vi "Teleop.vi"(10 "Match Info":T1={"Autonomous Elapsed Seconds"=0.0, "TeleOp Elapsed Seconds"=0.0, "Disabled Elapsed Seconds"=0.0, "Visited Autonomous"=FALSE, "Visited TeleOp"=FALSE, "Visited Disabled"=FALSE, "Autonomous Settings"={"Autonomous Style"=enum."Independent", "VI Refnum"=refnum}}, 11 "Call Context":T2) -> ()   [LabVIEW 2020]
doc: "This VI is called for each TeleOp packet received from the DS where the robot is not disabled. It is often used to read from the joysticks and update I/O or to update setpoints for timed control loops. It should complete and return within 20 milliseconds or it may miss DS packets."
uses:
  <vilib>/Rock Robotics/WPI/DriverStation/WPI_DriverStationDerivedRobotMode.ctl
  <vilib>/Rock Robotics/WPI/DriverStation/WPI_DriverStationMatch Info.ctl
  <vilib>/Rock Robotics/WPI/Joystick/XBox Buttons Indexer.ctl
  <vilib>/Rock Robotics/WPI/Joystick/XBox Axes Indexer.ctl
  <vilib>/Rock Robotics/WPI/Relay/WPI_RelayValue.ctl
  <vilib>/Rock Robotics/Network Tables/NT Read Boolean.vi
  <vilib>/Rock Robotics/Network Tables/NT Read Number.vi
  Auxilary/AuxGlobals.vi
  Climb/ClimbGlobals.vi
  <vilib>/Rock Robotics/Network Tables/NT Write String.vi
  Human/HumanGlobal.vi
  DriveSystem/DriveGlobals.vi
  <vilib>/Rock Robotics/Network Tables/NT Write Number.vi
  <vilib>/Rock Robotics/Network Tables/NT Write Boolean.vi
  Vision/VisionGlobals.vi
  <vilib>/Rock Robotics/WPI/Joystick/WPI_JoystickArcadeMapping.vi
  <vilib>/Rock Robotics/WPI/ThirdParty/JAS_Junk/TrajLib/Trajectory_Library.lvlib
panel:
  out "Sample Slider 0":dbl(slide) scale=0.0..5.0
  out "Sample Boolean 1":bool
  out "Sample Boolean 0":bool
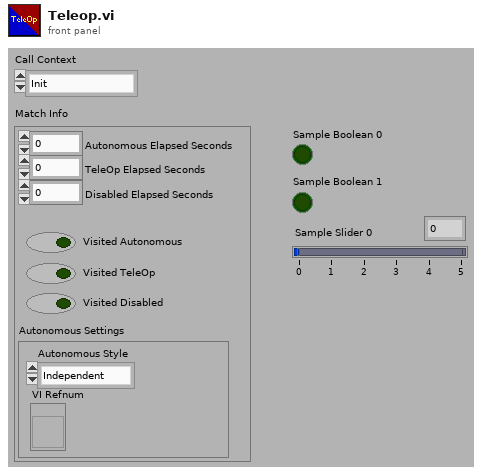
[diagram p1: front panel]
types:
  T1 = typedef "WPI_DriverStationMatch Info.ctl" = cluster{"Autonomous Elapsed Seconds":dbl, "TeleOp Elapsed Seconds":dbl, "Disabled Elapsed Seconds":dbl, "Visited Autonomous":bool, "Visited TeleOp":bool, "Visited Disabled":bool, "Autonomous Settings":cluster{"Autonomous Style":enum16{"Iterative", "Independent"}, "VI Refnum":refnum<vi>}}
  T2 = typedef "WPI_DriverStationDerivedRobotMode.ctl" = enum16{"Init", "Execute", "Stop"}
  T3 = typedef "XBox Buttons Indexer.ctl" = enum16{"A", "B", "X", "Y", "Left Bumper", "Right Bumper", "Back", "Start", "Left Joystick", "Right Joystick"}
  T4 = typedef "XBox Axes Indexer.ctl" = enum16{"Left X", "Left Y", "Left Trigger", "Right Trigger", "Right X", "Right Y"}
  T5 = typedef "WPI_RelayValue.ctl" = enum16{"Off", "On", "Forward", "Reverse"}
  T6 = typedef "WPI_RelayDevRef.ctl" = cluster{"DevStatus":errorcluster, "Relay Channel":T7, "Relay Direction":T8}
  T7 = typedef "FPGA_DIORelayChannel.ctl" = enum8{"Relay 0", "Relay 1", "Relay 2", "Relay 3", "Invalid"}
  T8 = typedef "WPI_RelayDirection.ctl" = enum16{"Both directions", "Forward only", "Reverse only"}
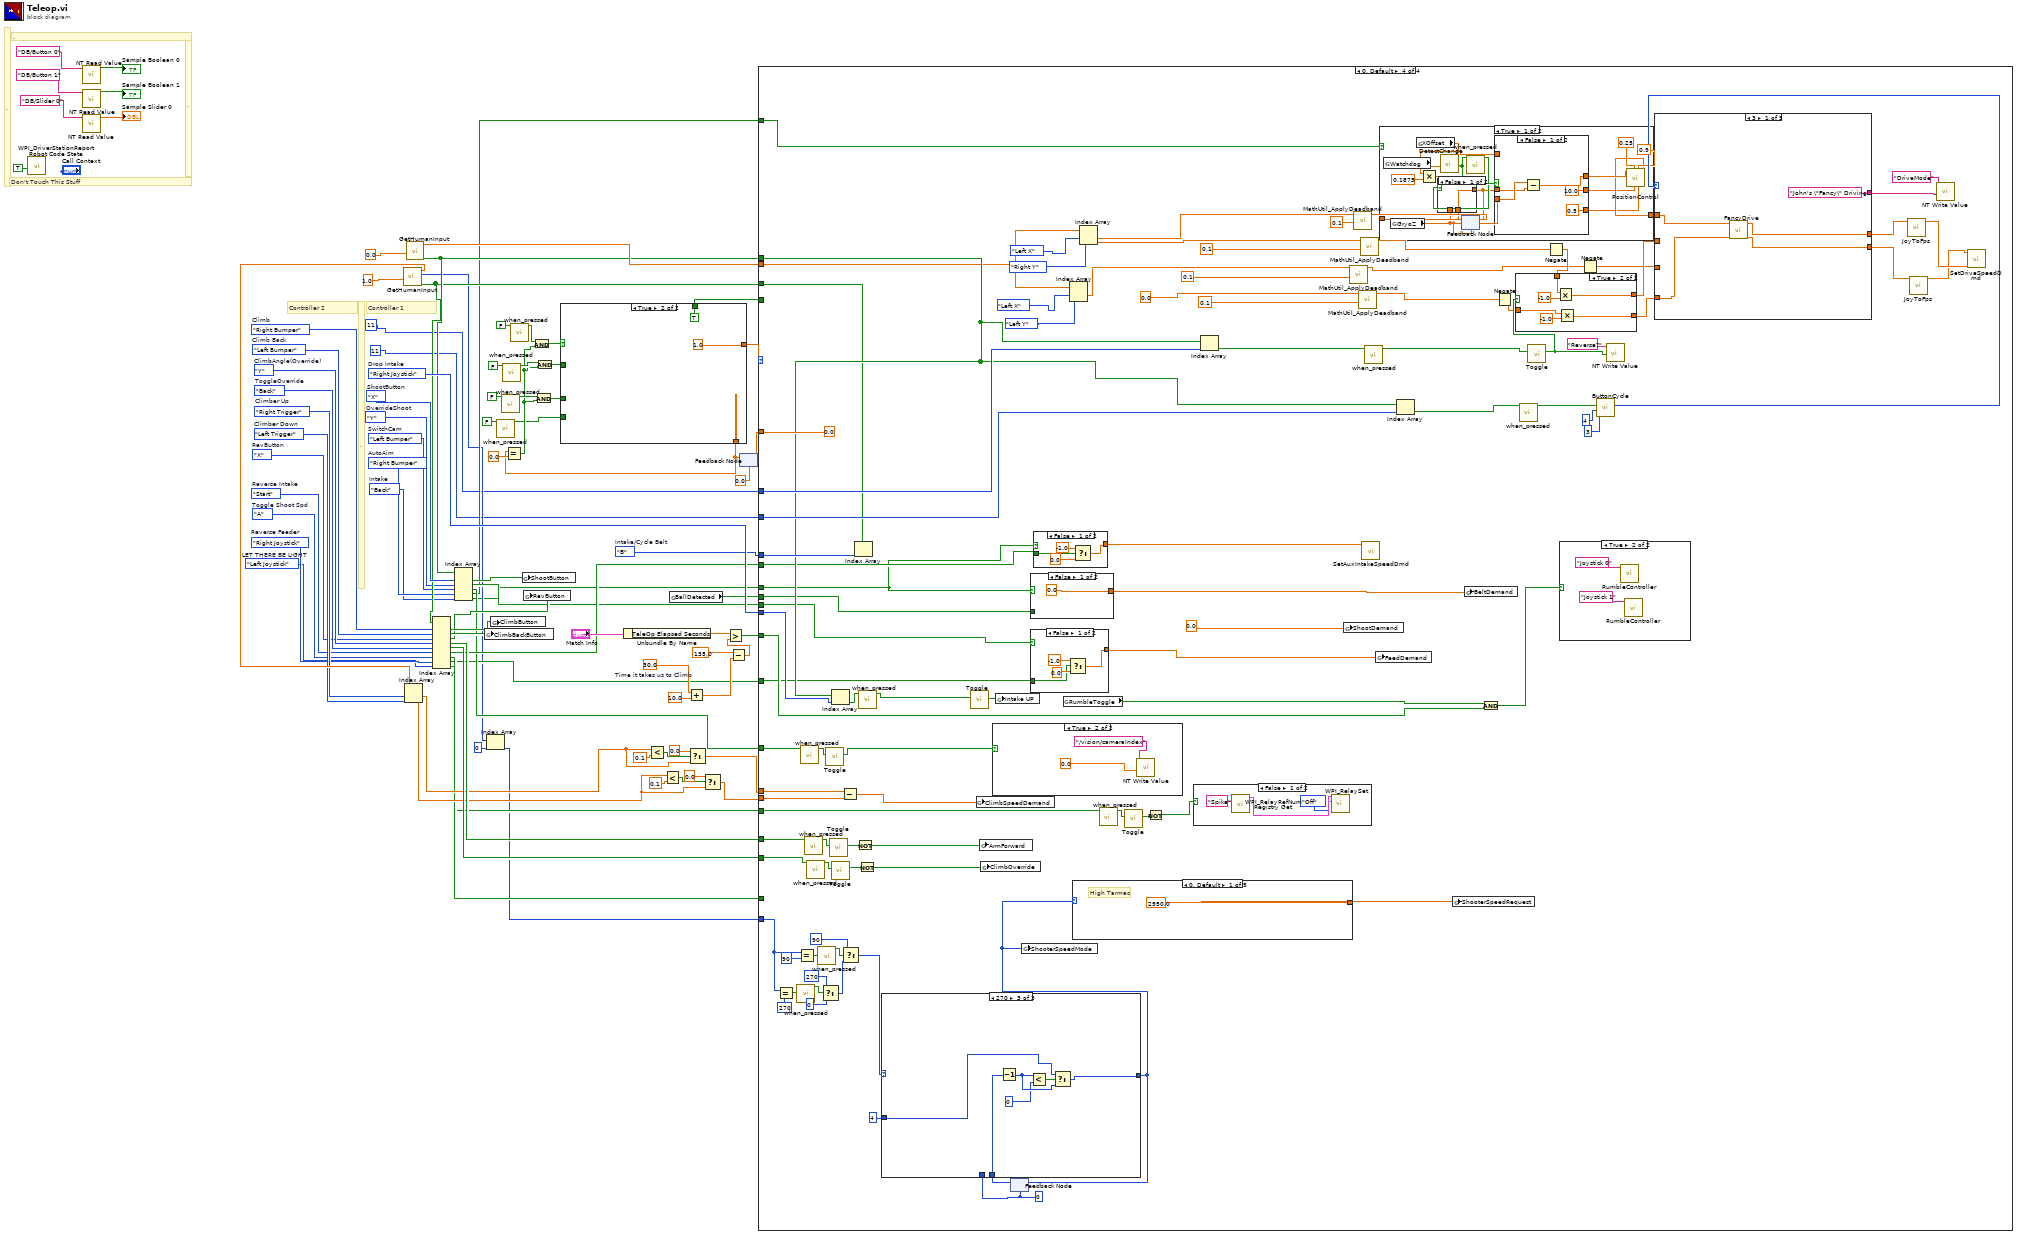
[diagram p0: block diagram]
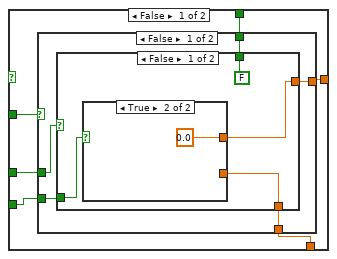
[diagram p2: hidden frame]
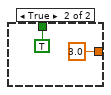
[diagram p4: hidden frame]
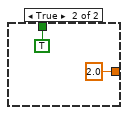
[diagram p5: hidden frame]
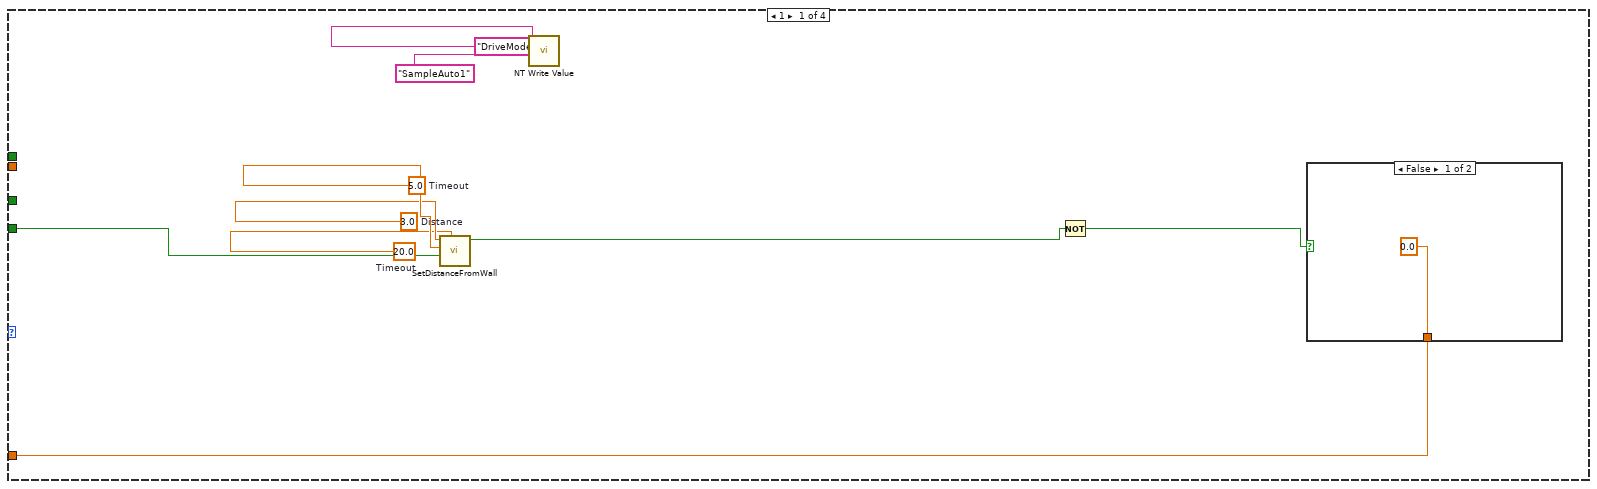
[diagram p6: hidden frame]
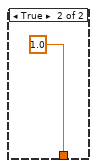
[diagram p7: hidden frame]
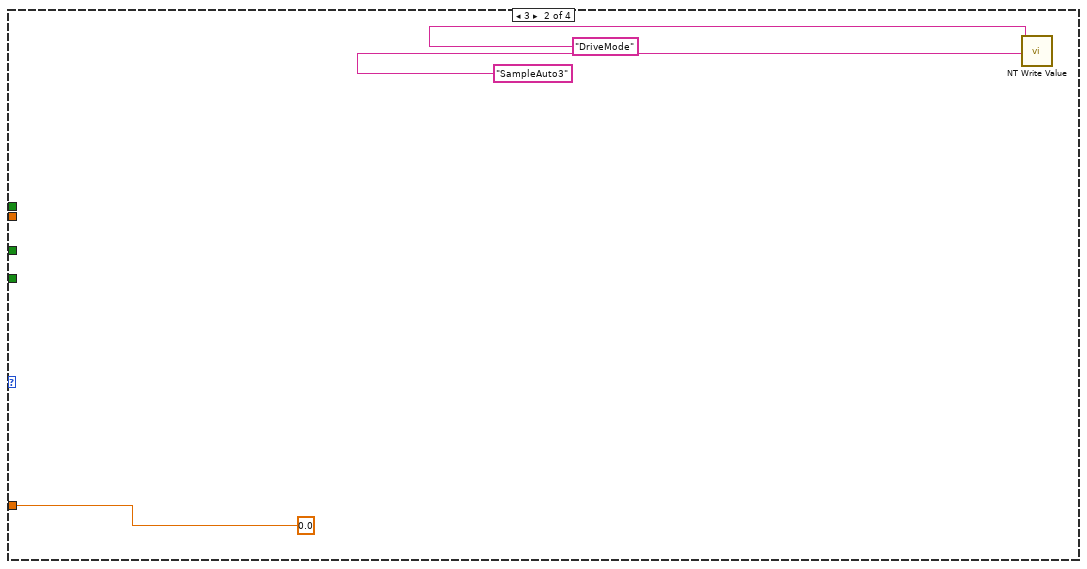
[diagram p8: hidden frame]
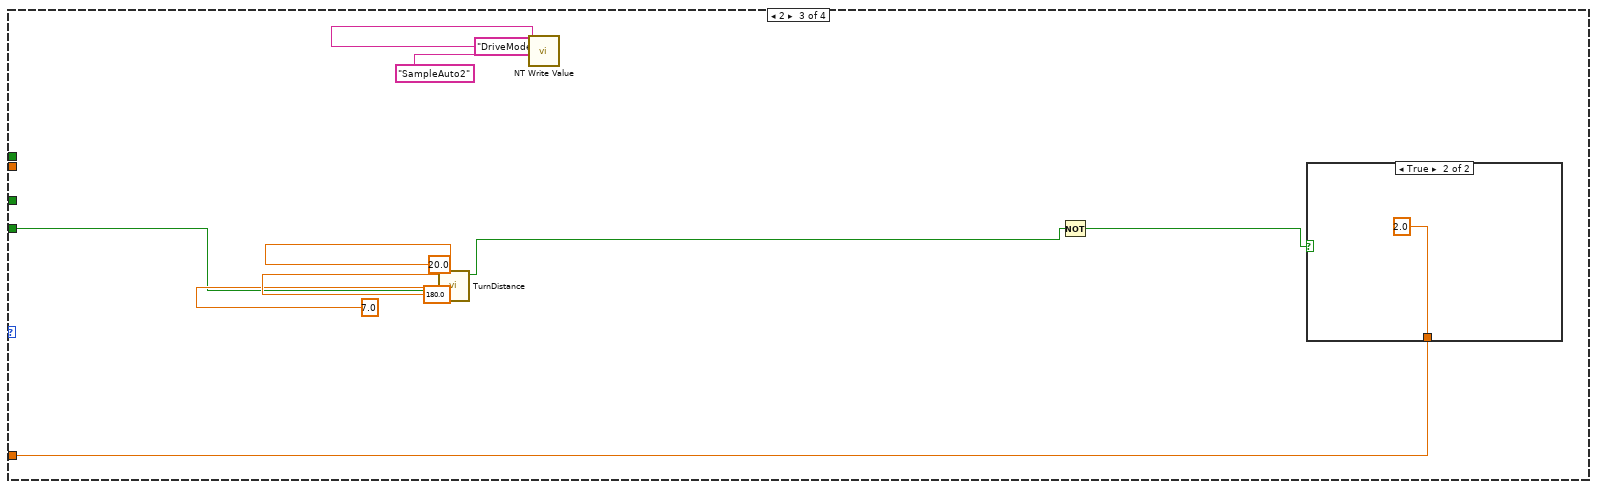
[diagram p9: hidden frame]
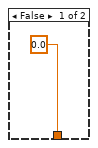
[diagram p10: hidden frame]
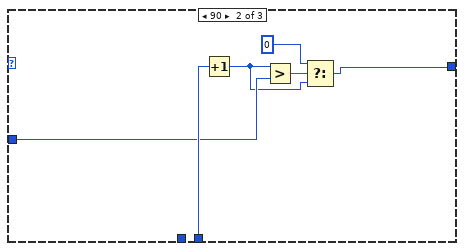
[diagram p12: hidden frame]
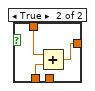
[diagram p13: hidden frame]
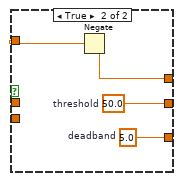
[diagram p14: hidden frame]
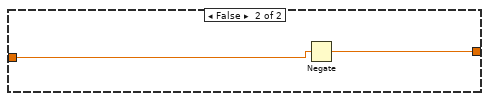
[diagram p15: hidden frame]
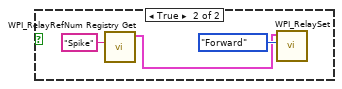
[diagram p16: hidden frame]
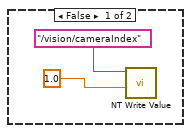
[diagram p17: hidden frame]
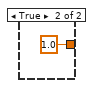
[diagram p18: hidden frame]
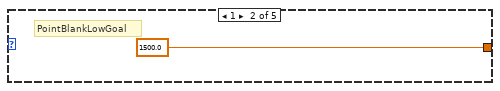
[diagram p19: hidden frame]
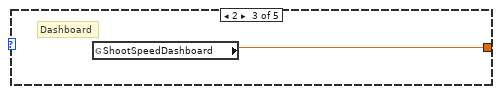
[diagram p20: hidden frame]
diagram:
  w2 = XBox_Buttons_Indexer."Back"  # Intake
  w10 = XBox_Buttons_Indexer."Right Bumper"  # AutoAim
  w12 = XBox_Buttons_Indexer."Left Joystick"  # LET THERE BE LIGHT
  w14 = XBox_Buttons_Indexer."Right Joystick"  # Reverse Feeder
  w16 = XBox_Buttons_Indexer."Left Bumper"  # SwitchCam
  w19 = XBox_Buttons_Indexer."Y"  # OverrideShoot
  w21 = XBox_Buttons_Indexer."A"  # Toggle Shoot Spd
  w33 = XBox_Buttons_Indexer."Start"  # Reverse Intake
  w42 = XBox_Buttons_Indexer."Left Bumper"  # Climb Back
  w43 = XBox_Axes_Indexer."Left Trigger"  # Climber Down
  w44 = XBox_Axes_Indexer."Right Trigger"  # Climber Up
  w47 = XBox_Buttons_Indexer."Back"  # ToggleOverride
  w48 = XBox_Buttons_Indexer."Y"  # ClimbAngle(Override)
  w52 = XBox_Buttons_Indexer."Right Bumper"  # Climb
  w54 = XBox_Buttons_Indexer."Right Joystick"  # Drop Intake
  w51 = XBox_Buttons_Indexer."B"  # Intake/Cycle Belt
  w62 = 30.0  # Time it takes us to Climb
  w36 = XBox_Buttons_Indexer."X"  # RevButton
  w56 = XBox_Buttons_Indexer."X"  # ShootButton
  # "."
  # "Controller 2"
  # "Controller 1"
  # "."
  # "."
  # "."
  # "Don't Touch This Stuff"
  n1 = call <vilib>:"WPI_DriverStationReport Robot Code State.vi"("TeleOp"=TRUE ("Autonomous")) -> ()  [unwired: 10 in, 1 out]
  n2 = call-poly <vilib>:"NT Read Value.vi"("Name"="DB/Button 0" ("refnum name")) -> ("Boolean"=→"Sample Boolean 0":bool)  [unwired: 9 in, 1 out]
  n3 = call-poly <vilib>:"NT Read Value.vi"("Name"="DB/Slider 0" ("refnum name")) -> ("Numeric"=→"Sample Slider 0":dbl)  [unwired: 9 in, 1 out]
  n4 = call-poly <vilib>:"NT Read Value.vi"("Name"="DB/Button 1" ("refnum name")) -> ("Boolean"=→"Sample Boolean 1":bool)  [unwired: 9 in, 1 out]
  n5 = call "GetHumanInput.vi"("Controller"=1.0) -> ("Buttons"=w34:bool[], "POVs"=w8:i16[], "Axes"=w45:dbl[])  [unwired: 8 in]
  n6 = Index Array(array=w45, index #1=w44, index #2=w43) -> (element #1=w29:dbl, element #2=w23:dbl)
  n7 = call "GetHumanInput.vi"("Controller"=0.0) -> ("Buttons"=w40:bool[], "Axes"=w79:dbl[])  [unwired: 8 in, 1 out]
  n8 = Index Array(array=w34, index #1=w52, index #2=w42, index #3=w36, index #4=w48, index #5=w47, index #6=w33, index #7=w21, index #8=w14, index #9=w12) -> (element #1=w53:bool, element #2=w41:bool, element #3=w35:bool, element #4=w49:bool, element #5=w46:bool, element #6=w32:bool, element #7=w20:bool, element #8=w13:bool, element #9=w11:bool)
  n9 = Index Array(array=w40, index #1=w56, index #2=w19, index #3=w16, index #4=w10, index #5=w2) -> (element #1=w57:bool, element #2=w18:bool, element #3=w15:bool, element #4=w9:bool, element #5=w3:bool)
  n10 = global write "ClimbGlobals.vi" "ClimbBackButton"(w41) -> ()
  n11 = Index Array(array=w8, index=0) -> (element=w6:i16)
  n12 = global write "ClimbGlobals.vi" "ClimbButton"(w53) -> ()
  n13 = call "when_pressed.vi"("Input"=FALSE) -> ("Output"=w65:bool)  [unwired: 10 in]
  n14 = call "when_pressed.vi"("Input"=FALSE) -> ("Output"=w69:bool)  [unwired: 10 in]
  n15 = call "when_pressed.vi"("Input"=FALSE) -> ("Output"=w68:bool)  [unwired: 10 in]
  n16 = call "when_pressed.vi"("Input"=FALSE) -> ("Output"=w72:bool)  [unwired: 10 in]
  n17 = global write "AuxGlobals.vi" "ShootButton"(w57) -> ()
  n18 = global write "AuxGlobals.vi" "RevButton"(w35) -> ()
  n19 = Unbundle By Name("Match Info") -> ("TeleOp Elapsed Seconds"=w64:dbl)
  n20 = Less?(x=w29, y=0.1) -> (x < y?=w30:bool)
  n21 = Less?(x=w23, y=0.1) -> (x < y?=w25:bool)
  n22 = global read "AuxGlobals.vi" "BallDetected"() -> (w50:bool)
  n23 = Add(x=w62, y=10.0) -> (x+y=w60:dbl)
  n24 = Select(t=0.0, s=w30, f=w29) -> (s? t:f=w27:dbl)
  n25 = Select(t=0.0, s=w25, f=w23) -> (s? t:f=w22:dbl)
  n26 = Subtract(x=135.0 ("y"), y=w60) -> (x-y=w59:dbl)
  n27 = Greater?(x=w64, y=w59) -> (0:w58:bool)
  n28 = feedback #1(0.0) -> (w74:dbl)
  n29 = Equal?(x=w74, y=0.0) -> (x = y?=w67:bool)
  n30 = And(x=w72, y=w67) -> (x .and. y?=w73:bool)
  n31 = And(x=w69, y=w67) -> (x .and. y?=w70:bool)
  n32 = And(x=w68, y=w67) -> (x .and. y?=w71:bool)
  n33 = case shown="True" w73 {
    tunnel: [w90 1.0] -> w17
    tunnel: w74 -> [w91 _]
    tunnel: w71 -> [w93 _]
    tunnel: w70 -> [w92 _]
    tunnel: [w89 TRUE] -> w66
    tunnel: w65 -> [w88 _]
    frame False {
      n34 = case shown="False" w93 {
        tunnel: w92 -> [w98 _]
        tunnel: w91 -> [w97 _]
        tunnel: [w96 2.0] -> w90
        tunnel: [w95 TRUE] -> w89
        tunnel: w88 -> [w94 _]
        frame False {
          n35 = case shown="False" w98 {
            tunnel: w97 -> [w99 _]
            tunnel: [w100 3.0] -> w96
            tunnel: [FALSE TRUE] -> w95
            tunnel: w94 -> [w101 _]
            frame False {
              n36 = case shown="True" w101 {
                tunnel: [w103 0.0] -> w100
                tunnel: w99 -> [w103 _]
                frame False {
                }
                frame True {
                }
              }
            }
            frame True {
            }
          }
        }
        frame True {
        }
      }
    }
    frame True {
    }
  }
  n37 = case shown="0, Default" w17 {
    tunnel: w79 -> [_ _ _ w182]
    tunnel: w40 -> [_ _ _ w199]
    tunnel: [w112 0.0 w130 0.0] -> w77
    tunnel: w66 -> [w111 _ w125 _]
    tunnel: 11 -> [_ _ _ w206]
    tunnel: 11 -> [_ _ _ w205]
    tunnel: w58 -> [_ _ _ w202]
    tunnel: w51 -> [_ _ _ w204]
    tunnel: w54 -> [_ _ _ w198]
    tunnel: w50 -> [_ _ _ w180]
    tunnel: w49 -> [_ _ _ w177]
    tunnel: w46 -> [_ _ _ w175]
    tunnel: w27 -> [_ _ _ w174]
    tunnel: w22 -> [_ _ _ w173]
    tunnel: w34 -> [_ _ _ w172]
    tunnel: w32 -> [_ _ _ w171]
    tunnel: w20 -> [_ _ _ _]
    tunnel: w18 -> [_ _ _ w164]
    tunnel: w15 -> [_ _ _ w161]
    tunnel: w13 -> [_ _ _ w160]
    tunnel: w11 -> [_ _ _ w156]
    tunnel: w9 -> [_ _ _ w155]
    tunnel: w6 -> [_ _ _ w140]
    tunnel: w3 -> [_ _ _ w137]
    frame 1 {
      w115 = 20.0  # Timeout
      w116 = 3.0  # Distance
      w117 = 5.0  # Timeout
      n38 = call "SetDistanceFromWall.vi"("Timeout"=w115, "Initation?"=w111, "MaxSpeed"=w117, "Distance"=w116) -> ("Finished"=w114:bool)  [unwired: 5 in, 2 out]
      n39 = call-poly <vilib>:"NT Write Value.vi"("String"="SampleAuto1", "Name"="DriveMode") -> ()  [unwired: 9 in, 1 out]
      n40 = Not(x=w114) -> (.not. x?=w113:bool)
      n41 = case shown="False" w113 {
        tunnel: [0.0 1.0] -> w112
        frame False {
        }
        frame True {
        }
      }
    }
    frame 3 {
      n42 = call-poly <vilib>:"NT Write Value.vi"("String"="SampleAuto3", "Name"="DriveMode") -> ()  [unwired: 9 in, 1 out]
    }
    frame 2 {
      n43 = call "TurnDistance.vi"("Timeout"=20.0, "Initation?"=w125, "MaxSpeed"=7.0, "Degrees"=180.0) -> ("Finished"=w129:bool)  [unwired: 5 in, 2 out]
      n44 = call-poly <vilib>:"NT Write Value.vi"("String"="SampleAuto2", "Name"="DriveMode") -> ()  [unwired: 9 in, 1 out]
      n45 = Not(x=w129) -> (.not. x?=w131:bool)
      n46 = case shown="True" w131 {
        tunnel: [0.0 2.0] -> w130
        frame False {
        }
        frame True {
        }
      }
    }
    frame 0, Default {
      w153 = 0
      n47 = Equal?(x=w140, y=i16 270) -> (x = y?=w147:bool)
      n48 = call "when_pressed.vi"("Input"=w147) -> ("Output"=w146:bool)  [unwired: 10 in]
      n49 = Equal?(x=w140, y=i16 90) -> (x = y?=w150:bool)
      n50 = call "when_pressed.vi"("Input"=w161) -> ("Output"=w163:bool)  [unwired: 10 in]
      n51 = call "when_pressed.vi"("Input"=w177) -> ("Output"=w178:bool)  [unwired: 10 in]
      n52 = call "when_pressed.vi"("Input"=w175) -> ("Output"=w176:bool)  [unwired: 10 in]
      n53 = call "when_pressed.vi"("Input"=w150) -> ("Output"=w149:bool)  [unwired: 10 in]
      n54 = Select(t=270, s=w146, f=0) -> (s? t:f=w142:i32)
      n55 = call "Toggle.vi"("FlashInput"=w163) -> ("On/Off"=w162:bool)  [unwired: 10 in]
      n56 = call "Toggle.vi"("FlashInput"=w178) -> ("On/Off"=w170:bool)  [unwired: 10 in]
      n57 = call "Toggle.vi"("FlashInput"=w176) -> ("On/Off"=w167:bool)  [unwired: 10 in]
      n58 = Index Array(array=w199, index=w198) -> (element=w196:bool)
      n59 = Subtract(x=w174, y=w173) -> (x-y=w181:dbl)
      n60 = Select(t=90, s=w149, f=w142) -> (s? t:f=w139:i32)
      n61 = Index Array(array=w172, index=w204) -> ()  [unwired: 1 out]
      n62 = Not(x=w170) -> (.not. x?=w169:bool)
      n63 = call "when_pressed.vi"("Input"=w196) -> ("Output"=w197:bool)  [unwired: 10 in]
      n64 = Not(x=w167) -> (.not. x?=w168:bool)
      n65 = call "Toggle.vi"("FlashInput"=w197) -> ("On/Off"=w200:bool)  [unwired: 10 in]
      n66 = global write "ClimbGlobals.vi" "ClimbSpeedDemand"(w181) -> ()
      n67 = global write "ClimbGlobals.vi" "ArmForward"(w169) -> ()
      n68 = global write "ClimbGlobals.vi" "ClimbOverride"(w168) -> ()
      n69 = case shown="True" w162 {
        frame False {
          n70 = call-poly <vilib>:"NT Write Value.vi"("Numeric"=1.0, "Name"="/vision/cameraIndex") -> ()  [unwired: 9 in, 1 out]
        }
        frame True {
          n71 = call-poly <vilib>:"NT Write Value.vi"("Numeric"=0.0, "Name"="/vision/cameraIndex") -> ()  [unwired: 9 in, 1 out]
        }
      }
      n72 = global write "AuxGlobals.vi" "Intake UP"(w200) -> ()
      n73 = feedback #2(w153) -> (w154:i32)
      n74 = case shown="270" w139 {
        tunnel: [w232 w233 w243] -> w151
        tunnel: w154 -> [w232 w238 w241]
        tunnel: w153 -> [_ _ _]
        tunnel: 4 ("MaxNum") -> [_ w236 w240]
        frame 0, Default {
        }
        frame 90 {
          n75 = Increment(x=w238) -> (x+1=w234:i32)
          n76 = Greater?(x=w234, y=w236) -> (0:w237:bool)
          n77 = Select(t=0, s=w237, f=w234) -> (s? t:f=w233:i32)
        }
        frame 270 {
          n78 = Decrement(x=w241) -> (x-1=w242:i32)
          n79 = Less?(x=w242, y=0) -> (x < y?=w244:bool)
          n80 = Select(t=w240, s=w244, f=w242) -> (s? t:f=w243:i32)
        }
      }
      n81 = feedback-in #2(w151) -> ()
      n82 = global write "AuxGlobals.vi" "ShooterSpeedMode"(w151) -> ()
      n83 = case shown="False" w137 {
        tunnel: [0.0 ("Shooter Demand") w302] -> w195
        tunnel: w180 -> [_ w300]
        frame False {
        }
        frame True {
          n84 = Select(t=0.0 ("Shooter Demand"), s=w300, f=0.8) -> (s? t:f=w302:dbl)
        }
      }
      n85 = case shown="False" w164 {
        tunnel: [w285 1.0 ("FeedDemand")] -> w165
        tunnel: w160 -> [w286 _]
        frame False {
          n86 = Select(t=-1.0, s=w286, f=0.0 ("FeedDemand")) -> (s? t:f=w285:dbl)
        }
        frame True {
        }
      }
      n87 = case shown="False" w137 {
        tunnel: [w304 1.0 ("Shooter Demand")] -> w136
        tunnel: w171 -> [w305 _]
        frame False {
          n88 = Select(t=-1.0, s=w305, f=0.0 ("Shooter Demand")) -> (s? t:f=w304:dbl)
        }
        frame True {
        }
      }
      n89 = global read "HumanGlobal.vi" "RumbleToggle"() -> (w203:bool)
      n90 = Index Array(array=w182, index #1=XBox_Axes_Indexer."Left X" ("XBox Axes"), index #2=XBox_Axes_Indexer."Left Y" ("XBox Axes")) -> (element #1=w185:dbl)  [unwired: 1 out]
      n91 = case shown="0, Default" w151 {
        tunnel: [2950.0 ("ShootSpeedDashboard") 1500.0 ("ShootSpeedDashboard") w292 w293 3500.0 ("ShootSpeedDashboard")] -> w166
        frame 0, Default {
          # "High Tarmac"
        }
        frame 1 {
          # "PointBlankLowGoal"
        }
        frame 2 {
          # "Dashboard"
          n92 = global read "AuxGlobals.vi" "ShootSpeedDashboard"() -> (w292:dbl)
        }
        frame 3 {
          # "HighGoalLidar"
          n93 = global read "DriveGlobals.vi" "LidarDistance"() -> (w297:dbl)
          n94 = Multiply(x=w297, y=98.0) -> (x*y=w295:dbl)
          n95 = Add(x=w295, y=2302.0) -> (x+y=w293:dbl)
        }
        frame 4 {
          # "LaunchPad"
        }
      }
      n96 = Index Array(array=w182, index #1=XBox_Axes_Indexer."Left X" ("XBox Axes"), index #2=XBox_Axes_Indexer."Right Y" ("XBox Axes")) -> (element #1=w191:dbl, element #2=w188:dbl)
      n97 = call "when_pressed.vi"("Input"=w156) -> ("Output"=w159:bool)  [unwired: 10 in]
      n98 = call "Toggle.vi"("FlashInput"=w159) -> ("On/Off"=w158:bool)  [unwired: 10 in]
      n99 = Not(x=w158) -> (.not. x?=w157:bool)
      n100 = case shown="False" w157 {
        frame False {
          n101 = call <vilib>:"WPI_RelayRefNum Registry Get.vi"("refnum name"="Spike") -> ("RelayDevRef"=w277:T6)  [unwired: 9 in, 1 out]
          n102 = call <vilib>:"WPI_RelaySet.vi"("RelayValue"=WPI_RelayValue."Off", "RelayDevRef"=w277) -> ()  [unwired: 8 in, 2 out]
        }
        frame True {
          n103 = call <vilib>:"WPI_RelayRefNum Registry Get.vi"("refnum name"="Spike") -> ("RelayDevRef"=w278:T6)  [unwired: 9 in, 1 out]
          n104 = call <vilib>:"WPI_RelaySet.vi"("RelayValue"=WPI_RelayValue."Forward", "RelayDevRef"=w278) -> ()  [unwired: 8 in, 2 out]
        }
      }
      n105 = Index Array(array=w199, index=w206) -> (element=w224:bool)
      n106 = global write "AuxGlobals.vi" "ShootDemand"(0.0 ("ShootDemand")) -> ()
      n107 = call <vilib>:"MathUtil_ApplyDeadband.vi"("Deadband"=0.1, "Value"=w185) -> ("Result"=w186:dbl)  [unwired: 9 in]
      n108 = call <vilib>:"MathUtil_ApplyDeadband.vi"("Deadband"=0.1, "Value"=w191) -> ("Result"=w192:dbl)  [unwired: 9 in]
      n109 = call <vilib>:"MathUtil_ApplyDeadband.vi"("Deadband"=0.1, "Value"=0.0) -> ("Result"=w183:dbl)  [unwired: 9 in]
      n110 = call <vilib>:"MathUtil_ApplyDeadband.vi"("Deadband"=0.1, "Value"=w188) -> ("Result"=w189:dbl)  [unwired: 9 in]
      n111 = call "SetAuxIntakeSpeedDmd.vi"("IntakeDemand"=w136) -> ()  [unwired: 11 in]
      n112 = call "when_pressed.vi"("Input"=w224) -> ("Output"=w222:bool)  [unwired: 10 in]
      n113 = global write "AuxGlobals.vi" "FeedDemand"(w165) -> ()
      n114 = case shown="True" w155 {
        tunnel: [w253 w274] -> w218
        tunnel: w192 -> [_ w273]
        frame True {
          n115 = global read "VisionGlobals.vi" "Watchdog"() -> (w259:dbl)
          n116 = global read "DriveGlobals.vi" "GryoZ"() -> (w247:dbl)
          n117 = global read "VisionGlobals.vi" "XOffset"() -> (w258:dbl)
          n118 = Multiply(x=w258, y=0.1875) -> (x*y=w250:dbl)
          n119 = call "DetectChange.vi"("Numeric"=w259) -> ("Boolean"=w252:bool)  [unwired: 10 in]
          n120 = feedback #3(w247) -> (w248:dbl)
          n121 = call "when_pressed.vi"("Input"=w252) -> ("Output"=w251:bool)  [unwired: 10 in]
          n122 = case shown="False" w251 {
            tunnel: w247 -> [_ w263]
            tunnel: w250 -> [_ w262]
            tunnel: [w260 w261] -> w249
            tunnel: w248 -> [w260 _]
            frame False {
            }
            frame True {
              n123 = Add(x=w262, y=w263) -> (x+y=w261:dbl)
            }
          }
          n124 = feedback-in #3(w249) -> ()
          n125 = case shown="False" w252 {
            tunnel: w258 -> [_ w272]
            tunnel: [w267 w271] -> w254
            tunnel: w247 -> [w268 _]
            tunnel: w249 -> [w266 _]
            tunnel: [10.0 ("threshold") w270] -> w246
            tunnel: [0.5 ("deadband") w269] -> w245
            frame False {
              n126 = Subtract(x=w268, y=w266) -> (x-y=w267:dbl)
            }
            frame True {
              w269 = 5.0  # deadband
              w270 = 50.0  # threshold
              n127 = Negate(x=w272) -> (-x=w271:dbl)
            }
          }
          n128 = call "PositionControl.vi"("deadband"=w245, "maxdemand"=0.9, "threshold"=w246, "mindemand"=0.25, "Error"=w254) -> ("output variable"=w253:dbl)  [unwired: 5 in, 1 out]
        }
        frame False {
          n129 = Negate(x=w273) -> (-x=w274:dbl)
        }
      }
      n130 = Index Array(array=w199, index=w205) -> (element=w230:bool)
      n131 = global write "AuxGlobals.vi" "ShooterSpeedRequest"(w166) -> ()
      n132 = global write "AuxGlobals.vi" "BeltDemand"(w195) -> ()
      n133 = And(x=w203, y=w202) -> (x .and. y?=w201:bool)
      n134 = Negate(x=w183) -> (-x=w215:dbl)
      n135 = call "when_pressed.vi"("Input"=w230) -> ("Output"=w214:bool)  [unwired: 10 in]
      n136 = call "Toggle.vi"("FlashInput"=w222) -> ("On/Off"=w220:bool)  [unwired: 10 in]
      n137 = Negate(x=w189) -> (-x=w217:dbl)
      n138 = case shown="True" w220 {
        tunnel: w217 -> [w313 w318]
        tunnel: w215 -> [w312 w316]
        tunnel: [w312 w315] -> w221
        tunnel: [w313 w314] -> w219
        frame False {
        }
        frame True {
          n139 = Multiply(x=w318, y=-1.0) -> (x*y=w314:dbl)
          n140 = Multiply(x=w316, y=-1.0) -> (x*y=w315:dbl)
        }
      }
      n141 = case shown="True" w201 {
        frame False {
          n142 = call "StopRumble.vi"("Controller Name"="Joystick 0") -> ()  [unwired: 11 in]
        }
        frame True {
          n143 = call "RumbleController.vi"("Controller Name"="Joystick 0") -> ()  [unwired: 11 in]
          n144 = call "RumbleController.vi"("Controller Name"="Joystick 1") -> ()  [unwired: 11 in]
        }
      }
      n145 = Negate(x=w186) -> (-x=w216:dbl)
      n146 = call "ButtonCycle.vi"("Start At"=3, "MaxNum"=4, "FlashInput"=w214) -> ("CycleNumber"=w213:i32)  [unwired: 8 in]
      n147 = call-poly <vilib>:"NT Write Value.vi"("Boolean"=w220, "Name"="Reverse?") -> ()  [unwired: 9 in, 1 out]
      n148 = case shown="3" w213 {
        tunnel: w216 -> [_ _ _ w343 _]
        tunnel: w221 -> [w322 w327 w337 w342 w344]
        tunnel: [w320 w328 w331 w341 w344] -> w229
        tunnel: [w321 w329 w330 w340 w345] -> w228
        tunnel: w218 -> [w323 w326 w338 _ _]
        tunnel: ["John's \"Fancy\" Driving" "Dual Arcade" "Precision" "Arcade" "Tank"] -> w225
        tunnel: w219 -> [_ _ _ _ w345]
        frame 3 {
          n149 = call "FancyDrive.vi"("Y axis value"=w322, "X axis value"=w323) -> ("Right Motor Value"=w321:dbl, "Left Motor Value"=w320:dbl)  [unwired: 8 in]
        }
        frame 1 {
          n150 = call-poly <vilib>:"WPI_JoystickMapping.vi"("Y axis value"=w327, "X axis value"=w326) -> ("Right Motor Value"=w329:dbl, "Left Motor Value"=w328:dbl)  [unwired: 8 in]
        }
        frame 2 {
          n151 = call-poly <vilib>:"WPI_JoystickMapping.vi"("Y axis value"=w337, "X axis value"=w338) -> ("Right Motor Value"=w335:dbl, "Left Motor Value"=w334:dbl)  [unwired: 8 in]
          n152 = Multiply(x=w334, y=0.5) -> (x*y=w331:dbl)
          n153 = Multiply(x=w335, y=0.5) -> (x*y=w330:dbl)
        }
        frame 0, Default {
          n154 = call-poly <vilib>:"WPI_JoystickMapping.vi"("Y axis value"=w342, "X axis value"=w343) -> ("Right Motor Value"=w340:dbl, "Left Motor Value"=w341:dbl)  [unwired: 8 in]
        }
        frame 4 {
        }
      }
      n155 = call "JoyToFps.vi"("JoystickInput"=w229) -> ("Fps"=w227:dbl)  [unwired: 10 in]
      n156 = call "JoyToFps.vi"("JoystickInput"=w228) -> ("Fps"=w226:dbl)  [unwired: 10 in]
      n157 = call-poly <vilib>:"NT Write Value.vi"("String"=w225, "Name"="DriveMode") -> ()  [unwired: 9 in, 1 out]
      n158 = call "SetDriveSpeedDmd.vi"("LeftSpeedInput"=w227, "RightSpeedInput"=w226) -> ()  [unwired: 10 in]
    }
  }
  n159 = feedback-in #1(w77) -> ()
